vi "Set pressed button flashing.vi"(8 "error in (no error)":errorcluster, 10 "Controll collection":T1) -> (0 "error out":errorcluster)   [LabVIEW 2011]
uses:
  Controll refrence groups.ctl
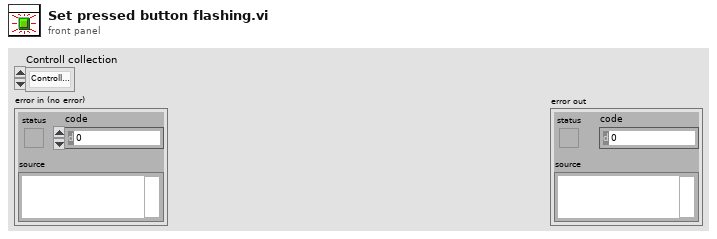
[diagram p1: front panel]
types:
  T1 = typedef "Controll refrence groups.ctl" = enum16{"Controller. gen", "Controller . High G", "Stroker", "PCP Online", "PCP Local", "PCP HV On", "Driller", "Stroker Cmd Buttons", "Stroker Anchor Cmd Buttons", "Controller Relay Buttons", "PCP Start Telemetry", "PCP Start Motor"}
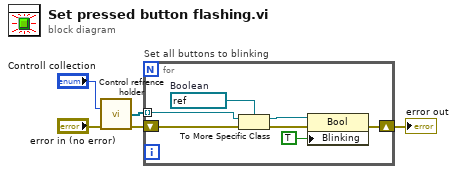
[diagram p0: block diagram]
diagram:
  n1 = call "Control refrence holder.vi"("Controll collection"="Controll collection", "error in (no error)"="error in (no error)") -> ("Controlls out"=w4:refnum<vi>[], "error out"=w3:errorcluster)  [unwired: 12 in]
  n2 = for "Set all buttons to blinking" {
    tunnel: w4 -> [w11] mode=indexing
    shift-right: [w6] -> w1
    shift-left: w3 -> [w8]
    w9 = refnum<vi> refnum  # Boolean
    n3 = To More Specific Class(target class=w9, reference=w11, error in=w8) -> (specific class reference=w10:refnum<vi>, error out=w7:errorcluster)
    n4 = property on="Property Node" class="Bool"(reference=w10, error in=w7, "Blinking"=TRUE) -> (error out=w6:errorcluster)  [unwired: 1 out]
  }
  "error out" <- w1
